vi "Lookup or Create Child.vi"(7 "Value Type (Object)":T1=enum."Object", 8 "error in (no error)":errorcluster, 10 "Name":string, 11 "Config Element in":refnum<class "Config Element.lvclass">) -> (0 "error out":errorcluster, 1 "Created New":bool, 2 "Child":refnum<class "Config Element.lvclass">, 3 "Config Element out":refnum<class "Config Element.lvclass">)   [LabVIEW 2023, in "CDM-Config.lvlib" / "Config Element.lvclass"]
doc: "Looks up a direct child by name. If the child does not exist a new one with the specified name is created."
uses:
  Config Element.lvclass
  Value Type.ctl
  Config Element.lvclass/Config Element.ctl
  CDM-Config.lvlib
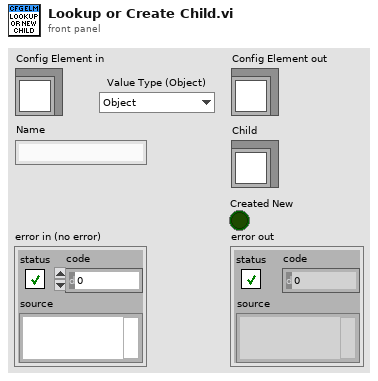
[diagram p1: front panel]
types:
  T1 = typedef "CDM-Config.lvlib/Value Type.ctl" = enum16{"String", "Number", "Bool", "Object", "Array"}
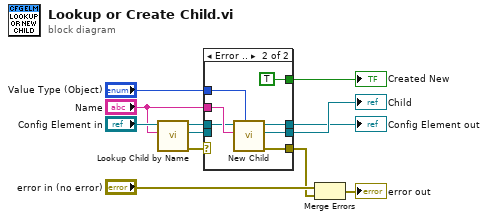
[diagram p0: block diagram]
diagram:
  n1 = call "Lookup Child by Name.vi"("Name"="Name", "Config Element in"="Config Element in") -> ("error out"=w5:errorcluster, "Child"=w1:refnum<class "Config Element.lvclass">, "Config Element out"=w2:refnum<class "Config Element.lvclass">)  [unwired: 6 in, 1 out]
  n2 = case shown="Error .." w5 {
    selector: w5 -> [w13 _]
    tunnel: w1 -> [w14 _]
    tunnel: w2 -> [w15 w21]
    tunnel: "Name" -> [_ w22]
    tunnel: [w15 w20] -> w7
    tunnel: [w14 w19] -> w8
    tunnel: [w13 w18] -> w6
    tunnel: [_ TRUE] -> w9
    tunnel: "Value Type (Object)" -> [_ w16]
    frame No Error {
    }
    frame Error {
      n3 = call "New Child.vi"("Value Type (Object)"=w16, "Child Name"=w22, "Config Element in"=w21) -> ("error out"=w18:errorcluster, "New Child"=w19:refnum<class "Config Element.lvclass">, "Config Element out"=w20:refnum<class "Config Element.lvclass">)  [unwired: 6 in]
    }
  }
  "Config Element out" <- w7
  "Child" <- w8
  "Created New" <- w9
  n4 = Merge Errors("error in (no error)", w6) -> (→"error out":errorcluster)
